vi "IsCommand.vi"(8 "error in (no error)":errorcluster, 11 "PathTokenizer in":refnum<class "PathTokenizer.lvclass">) -> (0 "error out":errorcluster, 2 "Is Command":bool, 3 "PathTokenizer out":refnum<class "PathTokenizer.lvclass">)   [LabVIEW 2019, in "PathTokenizer.lvclass"]
uses:
  PathTokenizer.lvclass
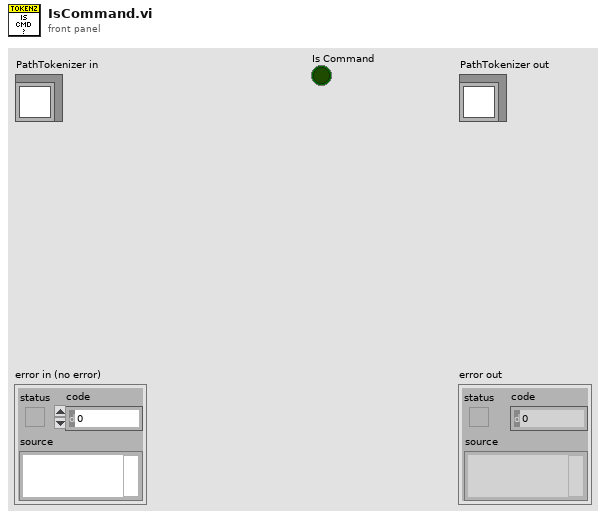
[diagram p1: front panel]
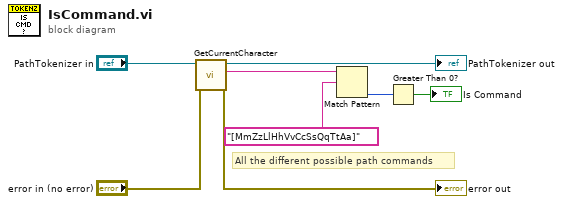
[diagram p0: block diagram]
diagram:
  # "All the different possible path commands"
  n1 = call "GetCurrentCharacter.vi"("error in (no error)"="error in (no error)", "PathTokenizer in"="PathTokenizer in") -> ("error out"=→"error out":errorcluster, "Current Character"=w4:string, "PathTokenizer out"=→"PathTokenizer out":refnum<class "PathTokenizer.lvclass">)  [unwired: 7 in]
  n2 = Match Pattern(string=w4, regular expression="[MmZzLlHhVvCcSsQqTtAa]") -> (offset past match=w2:i32)  [unwired: 1 in, 3 out]
  n3 = Greater Than 0?(x=w2) -> (x > 0?=→"Is Command":bool)
